vi "LVCAM Read LVCAM.vi"(11 "Self Actor in":refnum<class "Self Actor.lvclass">) -> (2 "LVCAM":refnum<class "LVCAM.lvclass">)   [LabVIEW 2021, in "LVCAM.lvlib" / "Self Actor.lvclass"]
uses:
  Self Actor.lvclass
  LVCAM/LVCAM.lvclass
  Self Actor.lvclass/Self Actor.ctl
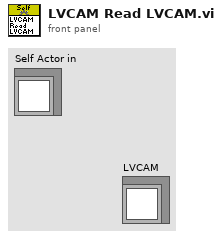
[diagram p1: front panel]
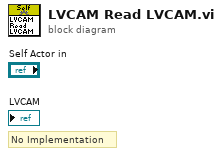
[diagram p0: block diagram]
diagram:
  # "No Implementation"
